vi "Pusher_Client_Connect.vi"(8 "ErrIn":errorcluster, 11 "Client in":refnum<class "Client.lvclass">) -> (0 "ErrOut":errorcluster, 2 "Reply":string, 3 "Client out":refnum<class "Client.lvclass">)   [LabVIEW 2009, in "Client.lvclass"]
uses:
  Client.lvclass
  Client.lvclass/Client.ctl
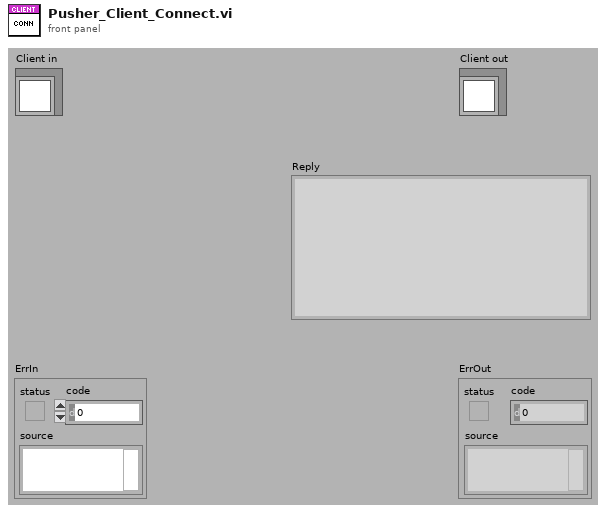
[diagram p1: front panel]
types:
  T1 = enum16{"Standard", "Buffered", "CRLF", "Immediate"}
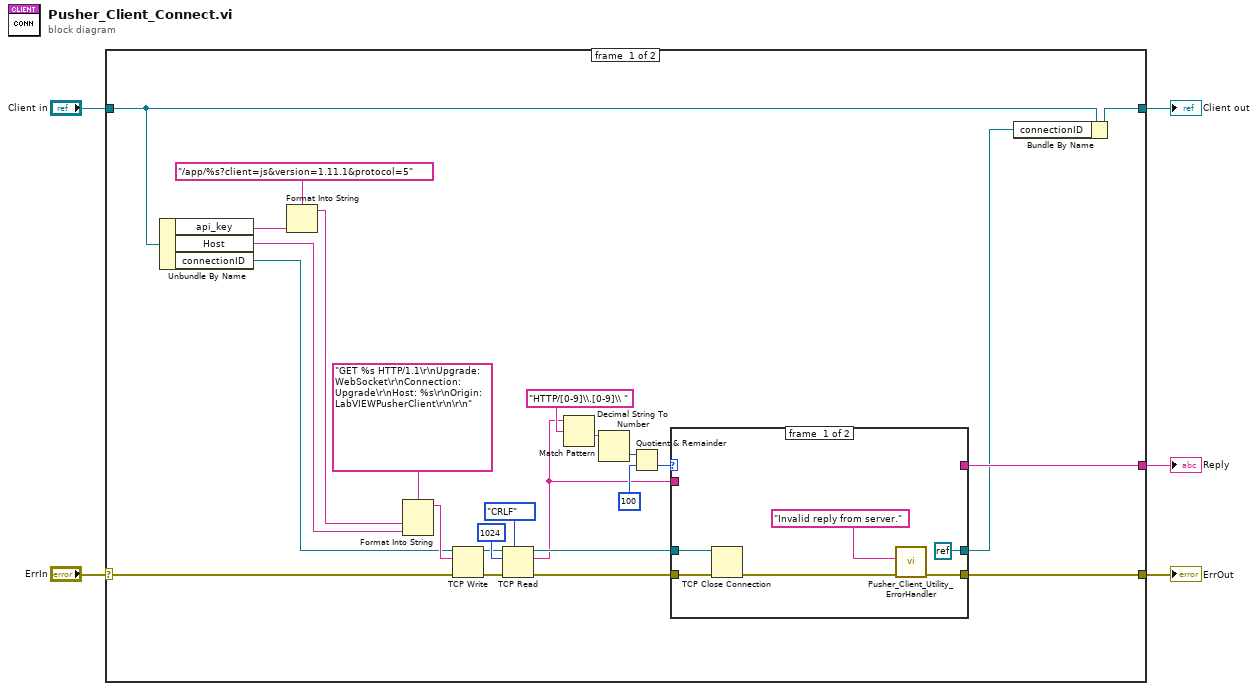
[diagram p0: block diagram]
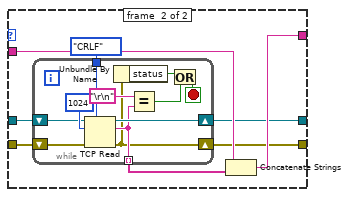
[diagram p2: hidden frame]
diagram:
  n1 = case shown="No Error" "ErrIn" {
    selector: "ErrIn" -> [w13 w57]
    tunnel: [w16 w57] -> w4
    tunnel: [w6 w56] -> w2
    tunnel: "Client in" -> [w9 w56]
    tunnel: [w10 _] -> w1
    frame #0 {
      n2 = Unbundle By Name(w9) -> ("api_key"=w14:string, "Host"=w12:string, "connectionID"=w11:refnum<k5>)
      n3 = Format Into String(format string="/app/%s?client=js&version=1.11.1&protocol=5", w14) -> (resulting string=w29:string)  [unwired: 2 in, 1 out]
      n4 = Format Into String(format string="GET %s HTTP/1.1\r\nUpgrade: WebSocket\r\nConnection: Upgrade\r\nHost: %s\r\nOrigin: LabVIEWPusherClient\r\n\r\n", w29, w12) -> (resulting string=w28:string)  [unwired: 2 in, 1 out]
      n5 = TCP Write(connection ID=w11, data in=w28, error in (no error)=w13) -> (connection ID out=w20:refnum<k5>, error out=w21:errorcluster)  [unwired: 1 in, 1 out]
      n6 = TCP Read(connection ID=w20, bytes to read=1024, error in (no error)=w21, 7:T1."CRLF" ("mode (standard)")) -> (connection ID out=w17:refnum<k5>, data out=w15:string, error out=w18:errorcluster)  [unwired: 1 in]
      n7 = Match Pattern(string=w15, regular expression="HTTP/[0-9]\\.[0-9]\\ ") -> (after substring=w24:string)  [unwired: 1 in, 3 out]
      n8 = Decimal String To Number(string=w24) -> (number=w22:i32)  [unwired: 2 in, 1 out]
      n9 = Quotient & Remainder(x=w22, y=100) -> (floor(x/y)=w19:i32)  [unwired: 1 out]
      n10 = case shown="1" w19 {
        tunnel: w18 -> [w36 w41]
        tunnel: w17 -> [w35 w42]
        tunnel: [w33 w38] -> w16
        tunnel: w15 -> [_ w40]
        tunnel: [_ w39] -> w10
        tunnel: [refnum<k0> refnum w37] -> w8
        frame #0 {
          n11 = TCP Close Connection(connection ID=w35, error in (no error)=w36) -> (error out=w34:errorcluster)  [unwired: 1 in, 1 out]
          n12 = call "Pusher_Client_Utility_ErrorHandler.vi"("ErrIn"=w34, "Additional Message"="Invalid reply from server.") -> ("ErrOut"=w33:errorcluster)  [unwired: 9 in]
        }
        frame #1 {
          n13 = while {
            tunnel: [w51] -> w44 mode=indexing
            tunnel: T1."CRLF" ("mode (standard)") -> [w53]
            shift-right: [w50] -> w38
            shift-left: w41 -> [w55]
            shift-right: [w54] -> w37
            shift-left: w42 -> [w45]
            stop <- w48 stop-if-true
            n14 = TCP Read(connection ID=w45, bytes to read=1024, error in (no error)=w55, 7:w53) -> (connection ID out=w54:refnum<k5>, data out=w51:string, error out=w50:errorcluster)  [unwired: 1 in]
            n15 = Unbundle By Name(w50) -> ("status"=w49:bool)
            n16 = Equal?(x="\r\n", y=w51) -> (x = y?=w47:bool)
            n17 = Or(x=w49, y=w47) -> (x .or. y?=w48:bool)
          }
          n18 = Concatenate Strings(w40, w44) -> (w39:string)
        }
      }
      n19 = Bundle By Name(cluster=w9, "connectionID"=w8) -> (w6:refnum<class "Client.lvclass">)
    }
    frame #1 {
    }
  }
  "ErrOut" <- w4
  "Client out" <- w2
  "Reply" <- w1
